vi "Motor_SetVolCmd.vi"(8 "error in (no error)":errorcluster, 10 "VolCmd":dbl[](array[numeric]), 11 "MotorCtrl in":refnum<class "MotorControl.lvclass">) -> (0 "error out":errorcluster, 2 "VolCmdOutput":dbl[](array[numeric]), 3 "MotorCtrl out":refnum<class "MotorControl.lvclass">)   [LabVIEW 2015, in "MotorControl.lvclass"]
uses:
  MotorControl.lvclass
  MotorControl.lvclass/MotorControl.ctl
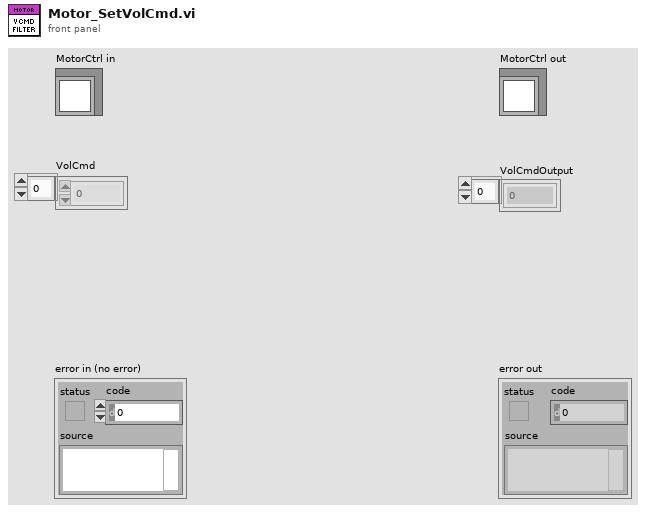
[diagram p1: front panel]
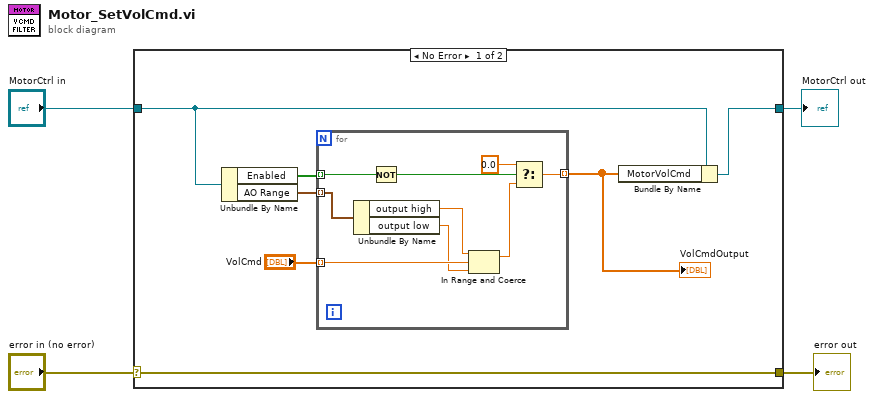
[diagram p0: block diagram]
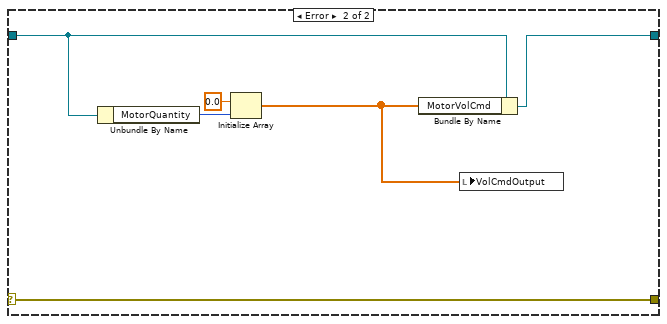
[diagram p2: hidden frame]
diagram:
  n1 = case shown="No Error" "error in (no error)" {
    selector: "error in (no error)" -> [w11 w26]
    tunnel: [w11 w26] -> w3
    tunnel: [w5 w22] -> w1
    tunnel: "MotorCtrl in" -> [w6 w23]
    frame No Error {
      n2 = Unbundle By Name(w6) -> ("Enabled"=w10:bool[], "AO Range"=w9:cluster{"output high":dbl, "output low":dbl}[])
      n3 = for {
        tunnel: w10 -> [w16] mode=indexing
        tunnel: w9 -> [w20] mode=indexing
        tunnel: "VolCmd" -> [w19] mode=indexing
        tunnel: [w13] -> w7 mode=indexing
        n4 = Unbundle By Name(w20) -> ("output high"=w18:dbl, "output low"=w17:dbl)
        n5 = Not(x=w16) -> (.not. x?=w12:bool)
        n6 = In Range and Coerce(upper limit=w18, x=w19, lower limit=w17) -> (coerced(x)=w15:dbl)  [unwired: 1 out]
        n7 = Select(t=0.0, s=w12, f=w15) -> (s? t:f=w13:dbl)
      }
      "VolCmdOutput" <- w7
      n8 = Bundle By Name(cluster=w6, "MotorVolCmd"=w7) -> (w5:refnum<class "MotorControl.lvclass">)
    }
    frame Error {
      n9 = Unbundle By Name(w23) -> ("MotorQuantity"=w25:i32)
      n10 = Initialize Array(0.0 ("element"), w25) -> (w21:dbl[])
      n11 = Bundle By Name(cluster=w23, "MotorVolCmd"=w21) -> (w22:refnum<class "MotorControl.lvclass">)
      n12 = local write "VolCmdOutput"(w21) -> ()
    }
  }
  "error out" <- w3
  "MotorCtrl out" <- w1
